vi "CronometroHMI.vi"() -> ()   [LabVIEW 2015]
uses:
  <vilib>/rvi/interface/nirviOpenFPGA/nirviOpenFPGA.xnode
  FPGA Bitfiles/final_FPGATarget_fpga_ehnNbasRIA0.lvbitx
  <vilib>/rvi/interface/nirviCloseFPGA/nirviCloseFPGA.xnode
  <vilib>/FPGAPlugInAG/Dynamic/niLvFpga_Close_Dynamic.vi
  <vilib>/FPGAPlugInAG/sbRIO-9636/niLvFpga_Open_sbRIO-9636.vi
  <vilib>/rvi/interface/common/dynamic/niFpgaDynamicAddResources.vi
panel:
  out ":":dbl
  out "?":dbl format="%_4f"
  out ":":dbl
  out ":":dbl
  out "Boolean 2":bool
  out "?":bool
  # "CRONOMETRO"
  # "SET"
  # "TIME"
  # "RESET"
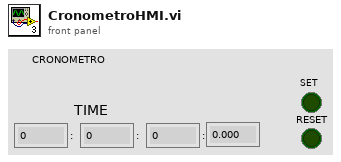
[diagram p1: front panel]
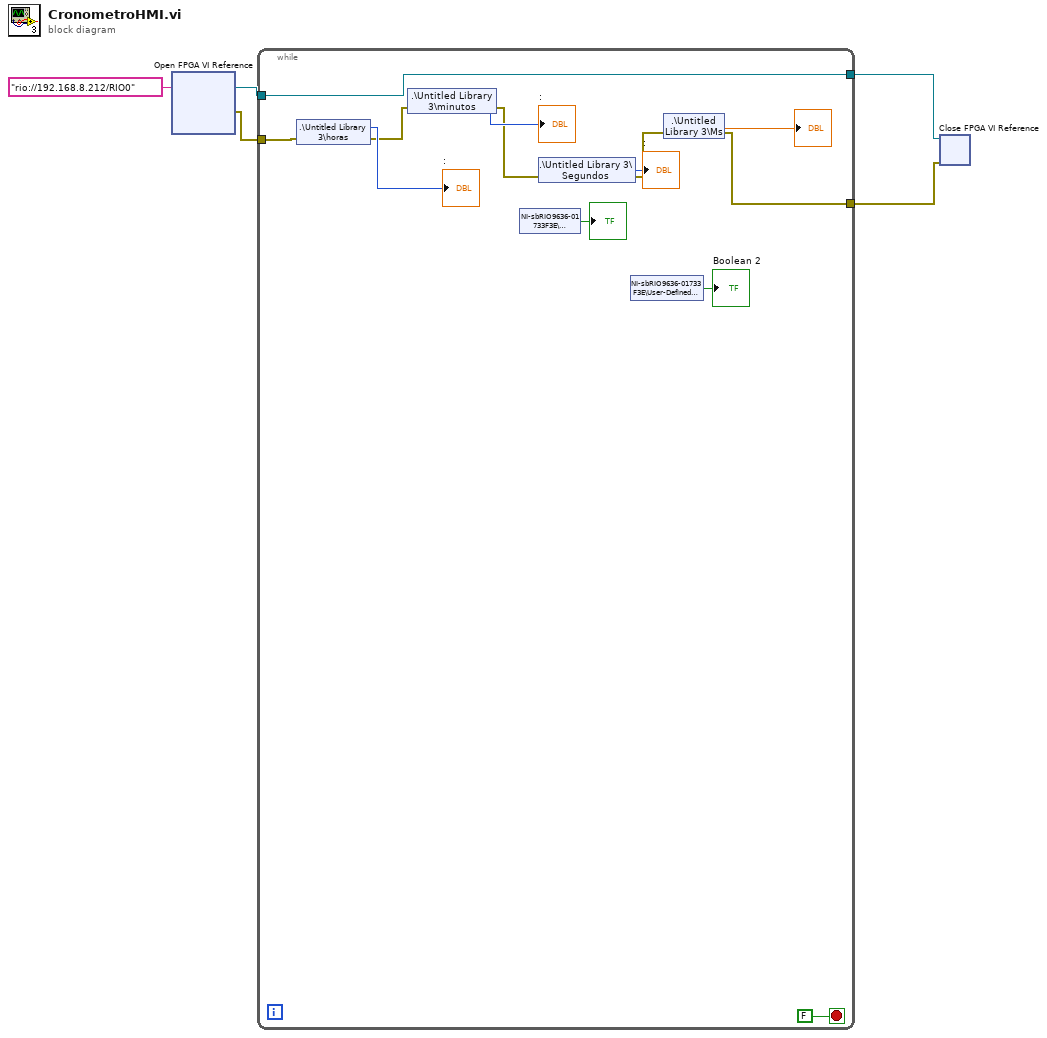
[diagram p0: block diagram]
diagram:
  n1 = xnode "Open FPGA VI Reference"("resource name"=tag "rio://192.168.8.212/RIO0") -> ("FPGA VI Reference Out"=w4:refnum<k20>, "error out"=w5:errorcluster)  [unwired: 1 in]
  n2 = while {
    tunnel: [w10] -> w3
    tunnel: w5 -> [w8]
    tunnel: w4 -> [w7]
    tunnel: [w7] -> w2
    stop <- FALSE stop-if-true
    n3 = shared-variable ".\\Untitled Library 3\\horas"(error in=w8) -> (→":":i16, error out=w9:errorcluster)
    n4 = shared-variable ".\\Untitled Library 3\\minutos"(error in=w9) -> (→":":i16, error out=w12:errorcluster)
    n5 = shared-variable "NI-sbRIO9636-01733F3E\\User-Defined Variables\\Set"() -> (→"?":bool)  [unwired: 1 in, 1 out]
    n6 = shared-variable ".\\Untitled Library 3\\Segundos"(error in=w12) -> (→":":i16, error out=w11:errorcluster)
    n7 = shared-variable "NI-sbRIO9636-01733F3E\\User-Defined Variables\\Reset"() -> (→"Boolean 2":bool)  [unwired: 1 in, 1 out]
    n8 = shared-variable ".\\Untitled Library 3\\Ms"(error in=w11) -> (→"?":dbl, error out=w10:errorcluster)
  }
  n9 = xnode "Close FPGA VI Reference"("FPGA VI Reference In"=w2, "error in"=w3) -> ()  [unwired: 1 out]
